vi "Fornax_Read Tester.vi"(10 "TCP Network Connection in":refnum<k5>, 11 "Cluster in":T1) -> (2 "TCP Network Connection out":refnum<k5>, 3 "Cluster out":T1)   [LabVIEW 2015]
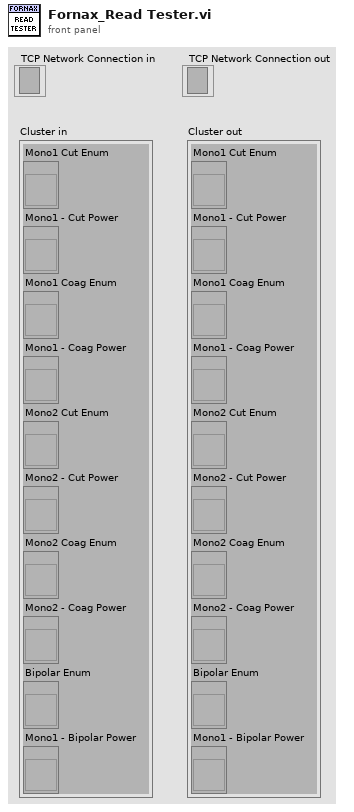
[diagram p1: front panel]
types:
  T1 = cluster{"Mono1 Cut Enum":refnum<vi>, "Mono1 - Cut Power":refnum<vi>, "Mono1 Coag Enum":refnum<vi>, "Mono1 - Coag Power":refnum<vi>, "Mono2 Cut Enum":refnum<vi>, "Mono2 - Cut Power":refnum<vi>, "Mono2 Coag Enum":refnum<vi>, "Mono2 - Coag Power":refnum<vi>, "Bipolar Enum":refnum<vi>, "Mono1 - Bipolar Power":refnum<vi>}
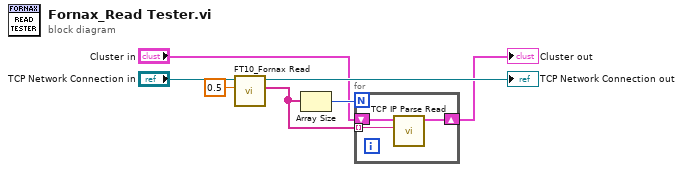
[diagram p0: block diagram]
diagram:
  n1 = call "FT10_Fornax Read.vi"("Timeout"=0.5, "TCP Network Connection in"="TCP Network Connection in") -> ("JSON Message"=w3:string[], "TCP Network Connection out"=→"TCP Network Connection out":refnum<k5>)  [unwired: 7 in, 1 out]
  n2 = Array Size(array=w3) -> (size(s)=w4:i32)
  n3 = for {
    N: w4 -> [_]
    tunnel: w3 -> [w10] mode=indexing
    shift-right: [w8] -> w5
    shift-left: "Cluster in" -> [w9]
    n4 = call "TCP IP Parse Read.vi"("JSON in"=w10, "Cluster in"=w9) -> ("Cluster out"=w8:T1)  [unwired: 8 in, 1 out]
  }
  "Cluster out" <- w5
